vi "testCheckListOfRegMsg.vi"(8 "error in (no error)":errorcluster) -> (0 "error out":errorcluster)   [LabVIEW 2018]
doc: "Test the checkListOfRegMsg.vi."
uses:
  src/TcpServer/TcpServer.lvclass
  src/TcpServer/TcpServer.lvclass/TcpServer.ctl
  src/TcpServerCmd/TcpServerCmd.lvclass
  home/pcortes/github/ts_labview_tcp_json/src/TcpServerBase/TcpServerBase.lvclass
  <vilib>/addons/_JKI Toolkits/Caraya/classes/Assert/Assert Equal Value_Variant.vi
  <vilib>/addons/_JKI Toolkits/Caraya/classes/Test/Test.lvclass
  <vilib>/addons/_JKI Toolkits/Caraya/classes/Assert/Assert.lvclass
  src/TcpServerBase/TcpServerBase.lvclass
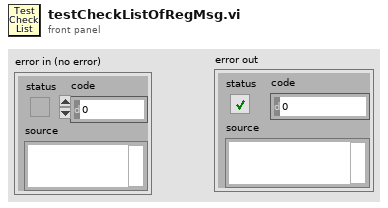
[diagram p1: front panel]
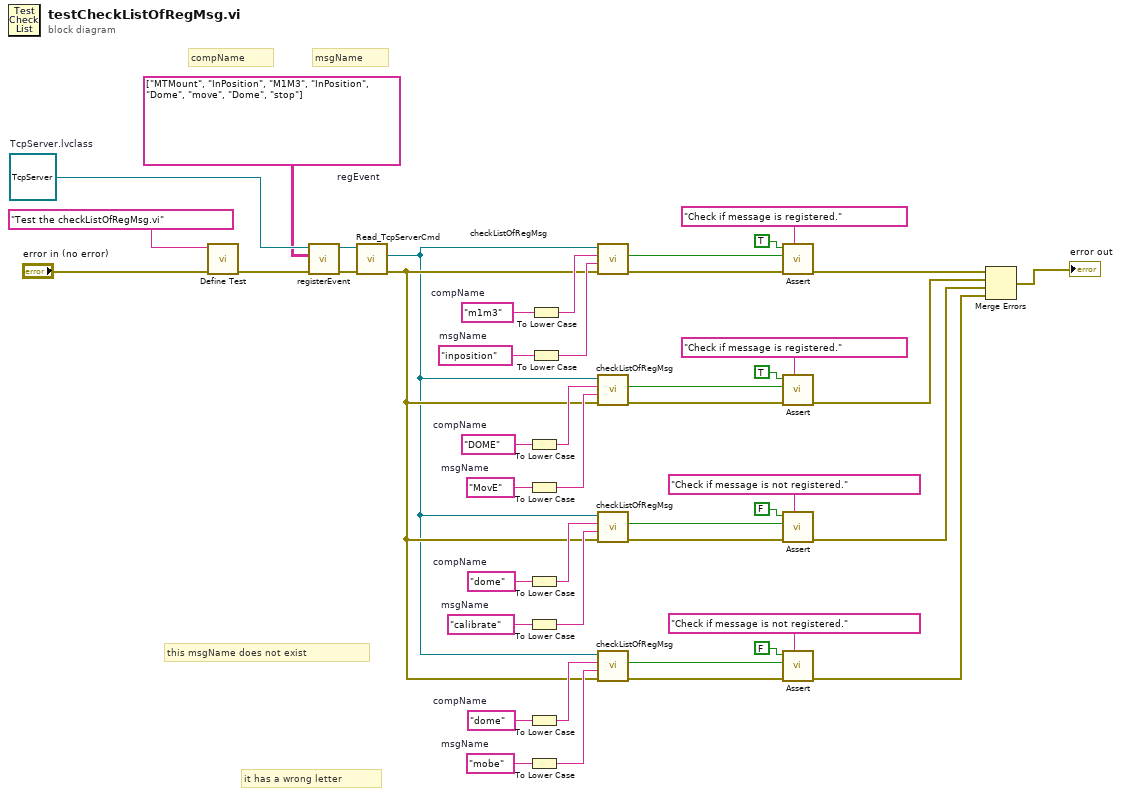
[diagram p0: block diagram]
diagram:
  w5 = "mobe"  # msgName
  w6 = "dome"  # compName
  w29 = "calibrate"  # msgName
  w28 = "dome"  # compName
  w30 = "MovE"  # msgName
  w31 = "DOME"  # compName
  w32 = "inposition"  # msgName
  w33 = "m1m3"  # compName
  w39 = string[][] [["MTMount", "InPosition"], ["M1M3", "InPosition"], ["Dome", "move"], ["Dome", "stop"]]  # regEvent
  w41 = refnum<class "TcpServer.lvclass"> refnum  # TcpServer.lvclass
  # "this msgName does not exist"
  # "it has a wrong letter"
  # "msgName"
  # "compName"
  n1 = call <vilib>:"Define Test.vi"("error in (no error)"="error in (no error)", "Label (VI Title)"="Test the checkListOfRegMsg.vi") -> ("error out"=w40:errorcluster)  [unwired: 9 in]
  n2 = call "registerEvent.vi"("error in (no error)"=w40, "regEvent"=w39, "tcpServer in"=w41) -> ("error out"=w38:errorcluster, "tcpServer out"=w37:refnum<class "TcpServer.lvclass">)  [unwired: 7 in]
  n3 = call "Read_TcpServerCmd.vi"("error in (no error)"=w38, "TcpServer in"=w37) -> ("error out"=w4:errorcluster, "TcpServerCmd.lvclass"=w3:refnum<class "TcpServerCmd.lvclass">)  [unwired: 7 in, 1 out]
  n4 = To Lower Case(string=w31) -> (all lower case string=w15:string)
  n5 = To Lower Case(string=w30) -> (all lower case string=w14:string)
  n6 = To Lower Case(string=w28) -> (all lower case string=w13:string)
  n7 = To Lower Case(string=w29) -> (all lower case string=w12:string)
  n8 = To Lower Case(string=w6) -> (all lower case string=w10:string)
  n9 = To Lower Case(string=w5) -> (all lower case string=w11:string)
  n10 = To Lower Case(string=w33) -> (all lower case string=w17:string)
  n11 = To Lower Case(string=w32) -> (all lower case string=w16:string)
  n12 = call "checkListOfRegMsg.vi"("error in (no error)"=w4, "msgName"=w16, "compName"=w17, "tcpServerBase in"=w3) -> ("error out"=w36:errorcluster, "msgRegistered?"=w35:bool)  [unwired: 5 in, 1 out]
  n13 = call "checkListOfRegMsg.vi"("error in (no error)"=w4, "msgName"=w14, "compName"=w15, "tcpServerBase in"=w3) -> ("error out"=w23:errorcluster, "msgRegistered?"=w22:bool)  [unwired: 5 in, 1 out]
  n14 = call "checkListOfRegMsg.vi"("error in (no error)"=w4, "msgName"=w12, "compName"=w13, "tcpServerBase in"=w3) -> ("error out"=w21:errorcluster, "msgRegistered?"=w20:bool)  [unwired: 5 in, 1 out]
  n15 = call "checkListOfRegMsg.vi"("error in (no error)"=w4, "msgName"=w11, "compName"=w10, "tcpServerBase in"=w3) -> ("error out"=w8:errorcluster, "msgRegistered?"=w9:bool)  [unwired: 5 in, 1 out]
  n16 = call-poly <vilib>:"Assert.vi"("Label"="Check if message is registered.", "error in (no error)"=w36, "Y"=w35, "X"=TRUE) -> ("error out"=w44:errorcluster)  [unwired: 7 in]
  n17 = call-poly <vilib>:"Assert.vi"("Label"="Check if message is registered.", "error in (no error)"=w23, "Y"=w22, "X"=TRUE) -> ("error out"=w19:errorcluster)  [unwired: 7 in]
  n18 = call-poly <vilib>:"Assert.vi"("Label"="Check if message is not registered.", "error in (no error)"=w21, "Y"=w20, "X"=FALSE) -> ("error out"=w18:errorcluster)  [unwired: 7 in]
  n19 = call-poly <vilib>:"Assert.vi"("Label"="Check if message is not registered.", "error in (no error)"=w8, "Y"=w9, "X"=FALSE) -> ("error out"=w2:errorcluster)  [unwired: 7 in]
  n20 = Merge Errors(w44, w19, w18, w2) -> (→"error out":errorcluster)
